vi "Receiver.vi"() -> ()   [LabVIEW 2019]
panel:
  out "Received":i32
  in  "stop":bool
  in  "address":string="127.0.0.1"
  in  "remote port":u16=3015
  out "Image":T1(plugin-control)
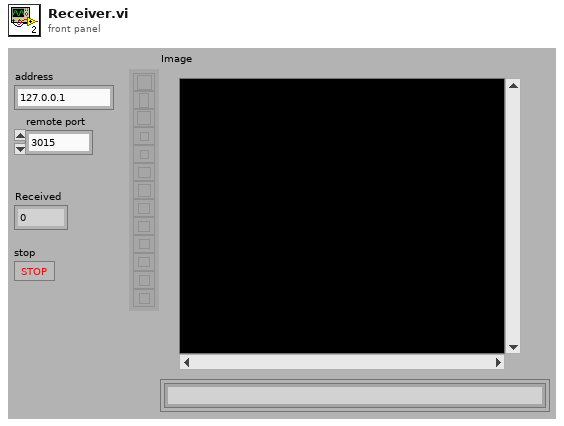
[diagram p1: front panel]
types:
  T1 = typedef "IMAQ Image.ctl" = refnum<image>
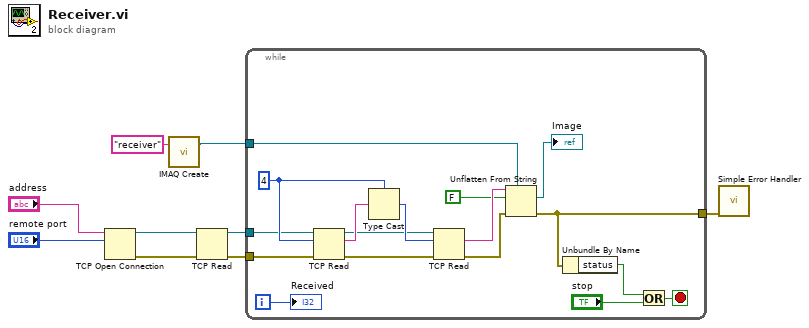
[diagram p0: block diagram]
diagram:
  n1 = TCP Open Connection(address="address", remote port or service name="remote port") -> (connection ID=w7:refnum<k5>, error out=w8:errorcluster)  [unwired: 3 in]
  n2 = call "IMAQ Create"("Image Name"="receiver") -> ("New Image"=w1:T1)  [unwired: 4 in, 1 out]
  n3 = TCP Read(connection ID=w7, error in (no error)=w8) -> (connection ID out=w3:refnum<k5>, error out=w4:errorcluster)  [unwired: 3 in, 1 out]
  n4 = while {
    tunnel: [w15] -> w9
    tunnel: w4 -> [w13]
    tunnel: w3 -> [w12]
    tunnel: w1 -> [w11]
    i -> [w10]
    stop <- w16 stop-if-true
    w22 = 4
    n5 = TCP Read(connection ID=w12, bytes to read=w22, error in (no error)=w13) -> (connection ID out=w24:refnum<k5>, data out=w26:string, error out=w23:errorcluster)  [unwired: 2 in]
    n6 = Type Cast(type=w22, x=w26) -> (*(type *) &x=w25:i32)
    n7 = TCP Read(connection ID=w24, bytes to read=w25, error in (no error)=w23) -> (data out=w21:string, error out=w18:errorcluster)  [unwired: 2 in, 1 out]
    n8 = Unflatten From String(type=w11, binary string=w21, data includes array or string size? (T)=FALSE, error in (no error)=w18) -> (value=→"Image":T1, error out=w15:errorcluster)  [unwired: 1 in, 1 out]
    n9 = Unbundle By Name(w15) -> ("status"=w14:bool)
    n10 = Or(x=w14, y="stop") -> (x .or. y?=w16:bool)
    "Received" <- w10
  }
  n11 = call <vilib>:"Simple Error Handler.vi"("error in (no error)"=w9) -> ()  [unwired: 4 in, 5 out]
